vi "ReadWrite Data.vi"(8 "error in":errorcluster, 9 "Read from VS Engine FIFO":refnum<k33>, 10 "Write to VS Engine FIFO":refnum<k33>, 11 "Channel Pairs":T2 {"Chan Refs" format="%.0x"}) -> (0 "error out":errorcluster, 2 "Read Occured":bool, 3 "Channel Pairs Out":T2 {"Chan Refs" format="%.0x"})   [LabVIEW 2013, in "Instrument Addon Engine.lvlib" / "Inline Async API.lvlib"]
uses:
  Inline Async API.lvlib
  <vilib>/NI Veristand/Custom Device API/Data Reference.ctl
  <vilib>/NI Veristand/Custom Device API/Global Data Refs.vi
  <vilib>/NI Veristand/Custom Device API/Custom Device API.lvlib
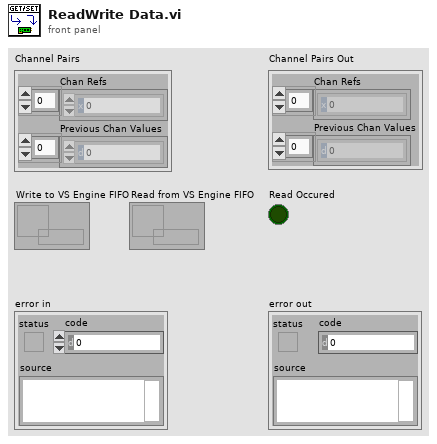
[diagram p1: front panel]
types:
  T1 = typedef "Custom Device API.lvlib/Data Reference.ctl" = i32
  T2 = cluster{"Chan Refs":T1[], "Previous Chan Values":dbl[]}
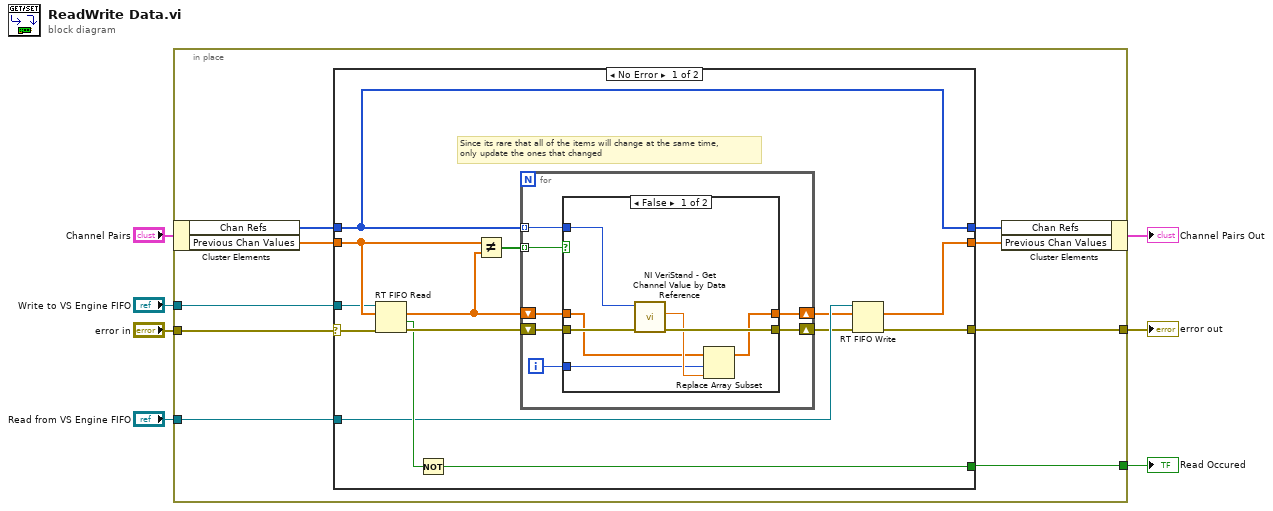
[diagram p0: block diagram]
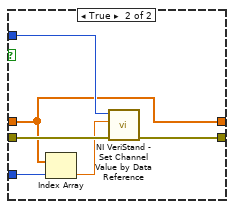
[diagram p2: hidden frame]
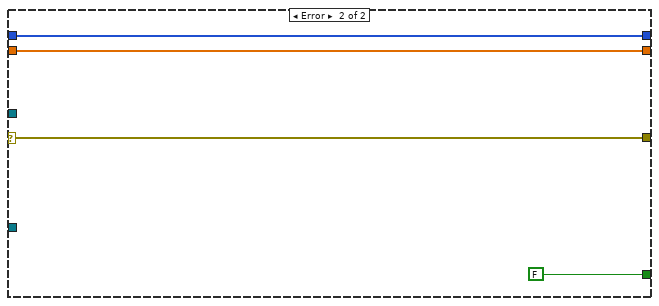
[diagram p3: hidden frame]
diagram:
  n1 = in-place {
    in-place-border: [w16] -> w7
    in-place-border: [w15] -> w6
    in-place-border: "error in" -> [w10]
    in-place-border: "Write to VS Engine FIFO" -> [w9]
    in-place-border: "Read from VS Engine FIFO" -> [w8]
    n2 = in-place-cluster #1("Channel Pairs") -> ("Chan Refs"=w14:T1[], "Previous Chan Values"=w13:dbl[])
    n3 = case shown="No Error" w10 {
      selector: w10 -> [w27 w53]
      tunnel: [w29 w53] -> w16
      tunnel: [w17 w51] -> w12
      tunnel: [w25 FALSE ("C Read Occured?")] -> w15
      tunnel: w14 -> [w22 w50]
      tunnel: w13 -> [w24 w51]
      tunnel: [w22 w50] -> w11
      tunnel: w9 -> [w21 _]
      tunnel: w8 -> [w20 _]
      frame No Error {
        # "Since its rare that all of the items will change at the same time,\nonly update the ones that changed"
        n4 = RT FIFO Read(0:w21, 1:w24, 3:w27) -> (9:w23:dbl[], 10:w26:bool, 11:w28:errorcluster)  [unwired: 1 in, 2 out]
        n5 = Not(x=w26) -> (.not. x?=w25:bool)
        n6 = Not Equal?(x=w24, y=w23) -> (x != y?=w19:bool[])
        n7 = for {
          shift-right: [w36] -> w18
          shift-left: w28 -> [w35]
          tunnel: w19 -> [w32] mode=indexing
          tunnel: w22 -> [w33] mode=indexing
          shift-right: [w30] -> w17
          shift-left: w23 -> [w34]
          i -> [w31]
          n8 = case shown="False" w32 {
            tunnel: w34 -> [w38 w44]
            tunnel: [w41 w48] -> w36
            tunnel: w35 -> [w42 w49]
            tunnel: w33 -> [w43 w47]
            tunnel: w31 -> [w39 w46]
            tunnel: [w37 w44] -> w30
            frame False {
              n9 = call <vilib>:"NI VeriStand - Get Channel Value by Data Reference.vi"("error in (no error)"=w42, "Data Reference in"=w43) -> ("error out"=w41:errorcluster, "Value"=w40:dbl)  [unwired: 8 in]
              n10 = Replace Array Subset(array=w38, new element=w40, index=w39) -> (w37:dbl[])
            }
            frame True {
              n11 = Index Array(array=w44, index=w46) -> (element=w45:dbl)
              n12 = call <vilib>:"NI VeriStand - Set Channel Value by Data Reference.vi"("error in (no error)"=w49, "Value"=w45, "Data Reference in"=w47) -> ("error out"=w48:errorcluster)  [unwired: 8 in]
            }
          }
        }
        n13 = RT FIFO Write(0:w20, 1:w17, 3:w18) -> (11:w29:errorcluster)  [unwired: 2 in, 3 out]
      }
      frame Error {
      }
    }
    n14 = in-place-cluster #1("Chan Refs"=w11, "Previous Chan Values"=w12) -> (→"Channel Pairs Out":T2)
  }
  "error out" <- w7
  "Read Occured" <- w6
